vi "LWXPS_DebugServitudesTimeUsageGet.vi"(0 "XPS Reference IN":refnum<k24>, 5 "LabVIEW error IN":errorcluster) -> (12 "XPS Reference OUT":refnum<k24>, 13 "LabVIEW error OUT":errorcluster, 14 "Returned error code":i32, 15 "ISR Profile Servitudes Delta":dbl, 16 "ISR Error Check Duration":dbl, 17 "ISR Groups Duration":dbl, 18 "ISR Init Param Duration":dbl, 19 "XPS Error String":string)   [LabVIEW 2014]
uses:
  D:/XPSQ8_LabView_Library/Development/Source/Dll/Newport.XPS.CommandInterface.dll
  Dll/Newport.XPS.CommandInterface.dll
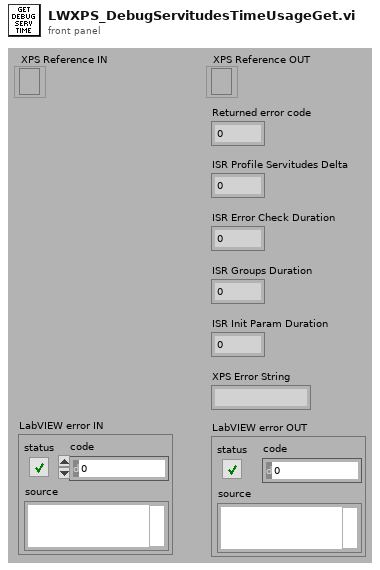
[diagram p1: front panel]
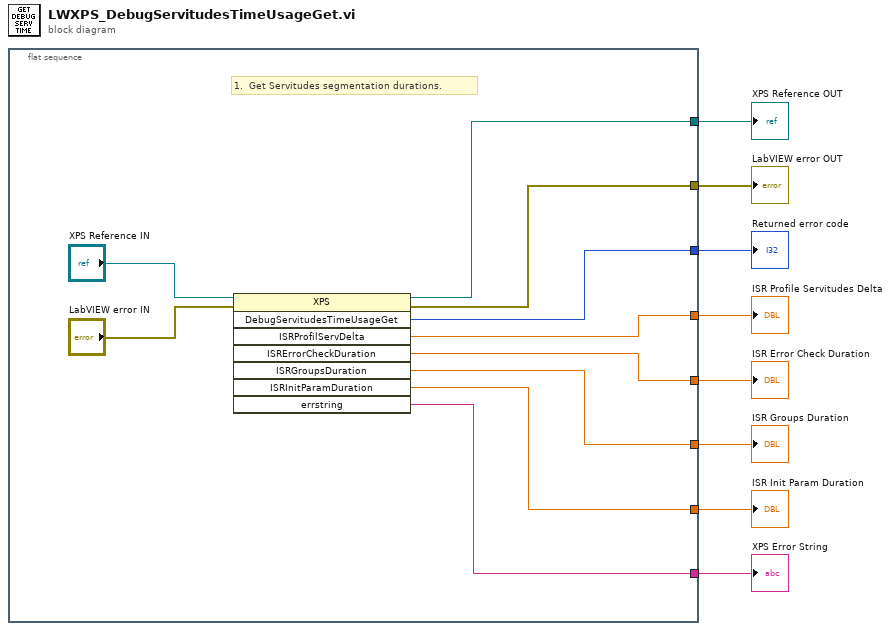
[diagram p0: block diagram]
diagram:
  n1 = flat-sequence {
    tunnel: [w16] -> w8
    tunnel: [w14] -> w7
    tunnel: [w17] -> w6
    tunnel: [w13] -> w4
    tunnel: [w12] -> w3
    tunnel: [w11] -> w5
    tunnel: [w10] -> w1
    tunnel: [w9] -> w2
    frame #0 {
      # "1.  Get Servitudes segmentation durations."
      n2 = invoke class="XPS" method="DebugServitudesTimeUsageGet"(reference="XPS Reference IN", error in="LabVIEW error IN") -> (reference out=w16:refnum<k24>, error out=w14:errorcluster, "DebugServitudesTimeUsageGet"=w17:i32, "ISRProfilServDelta"=w11:dbl, "ISRErrorCheckDuration"=w13:dbl, "ISRGroupsDuration"=w12:dbl, "ISRInitParamDuration"=w10:dbl, "errstring"=w9:string)  [unwired: 6 in]
    }
  }
  "XPS Reference OUT" <- w8
  "LabVIEW error OUT" <- w7
  "Returned error code" <- w6
  "XPS Error String" <- w2
  "ISR Profile Servitudes Delta" <- w5
  "ISR Error Check Duration" <- w4
  "ISR Groups Duration" <- w3
  "ISR Init Param Duration" <- w1
